vi "Class - By Folder.vi"(7 "Msg Chain":string, 8 "error in (no error)":errorcluster {"code" format="Error %.0f"}, 10 "Classes":refnum<class "Class Documentation.lvclass">[](array[class]), 11 "VIDoc Printer In":refnum<class "VIDoc Printer.lvclass">) -> (0 "error out":errorcluster {"code" format="Error %.0f"}, 3 "VIDoc Printer Out":refnum<class "VIDoc Printer.lvclass">)   [LabVIEW 2023, in "VIDoc Printer.lvlib" / "VIDoc Printer.lvclass"]
uses:
  VIDoc Printer.lvclass
  Parsing/Class Documentation/Class Documentation.lvclass
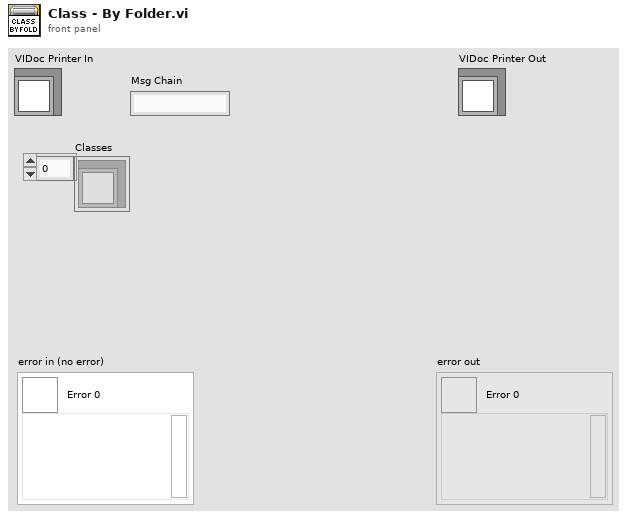
[diagram p1: front panel]
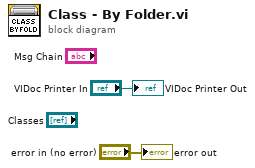
[diagram p0: block diagram]
diagram:
  "error out" <- "error in (no error)"
  "VIDoc Printer Out" <- "VIDoc Printer In"
